vi "计算结果-开启关闭.vi"(5 "油动机试验路径":path=path "D:/研究生/课程/油动机项目/实验文件夹/168-15-6201-004/GV2") -> (0 "计算参数 out":T1, 1 "输入参数":T2, 2 "开启关闭试验":cluster{dbl, dbl, dbl[][]}(graph))   [LabVIEW 2013]
uses:
  <vilib>/Analysis/3filter.llb/Filter Passband Type.ctl
  <vilib>/Utility/config.llb/Read Key (String).vi
  <vilib>/Analysis/3filter.llb/Butterworth Filter (DBL).vi
  <vilib>/Analysis/NI_AALBase.lvlib
  <vilib>/Utility/config.llb/NI_LVConfig.lvlib
panel:
  in  "计算参数 in":T1
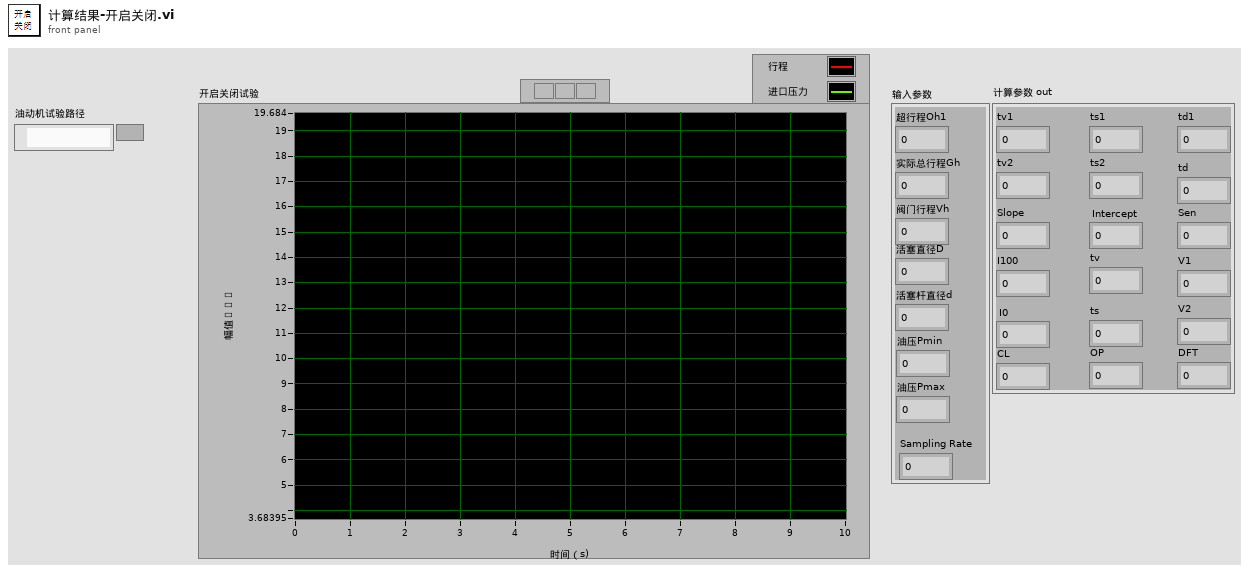
[diagram p1: front panel]
types:
  T1 = cluster{"tv1":dbl, "tv2":dbl, "tv":dbl, "ts1":dbl, "ts2":dbl, "ts":dbl, "td1":dbl, "td":dbl, "Slope":dbl, "Intercept":dbl, "I100":dbl, "I0":dbl, "Sen":dbl, "V1":dbl, "V2":dbl, "CL":dbl, "OP":dbl, "DFT":dbl}
  T2 = cluster{"超行程Oh1":dbl, "实际总行程Gh":dbl, "阀门行程Vh":dbl, "活塞直径D":dbl, "活塞杆直径d":dbl, "油压Pmin":dbl, "油压Pmax":dbl, "Sampling Rate":dbl}
  T3 = typedef "NI_AALBase.lvlib/Filter Passband Type.ctl" = enum32{"Lowpass", "Highpass", "Bandpass", "Bandstop"}
  T4 = typedef "NI_LVConfig.lvlib/Config Data RefNum.ctl" = refnum<k1>
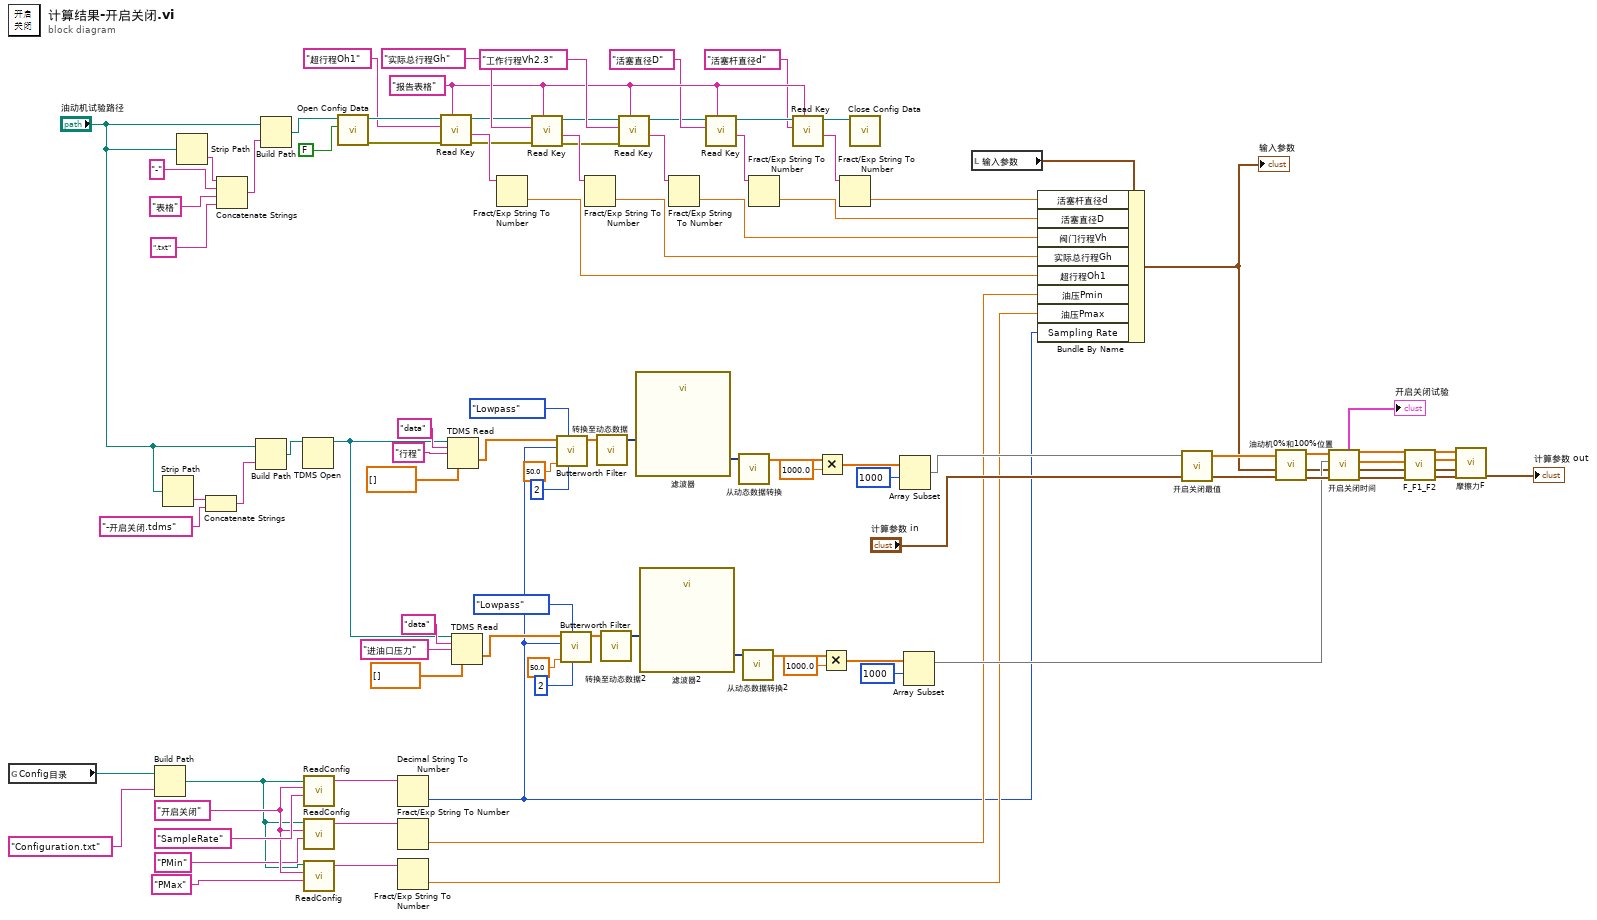
[diagram p0: block diagram]
diagram:
  w17 = "开启关闭" ("Section")
  w54 = "报告表格" ("key")
  n1 = global read "Config目录.vi" "Config目录"() -> (w20:path)
  n2 = Build Path(base path=w20, name or relative path="Configuration.txt") -> (appended path=w14:path)
  n3 = Strip Path(path="油动机试验路径") -> (name=w64:string)  [unwired: 1 out]
  n4 = Strip Path(path="油动机试验路径") -> (name=w61:string)  [unwired: 1 out]
  n5 = Concatenate Strings(w64, "-开启关闭.tdms") -> (w62:string)
  n6 = Concatenate Strings(w61, "-" ("string"), "表格" ("string"), ".txt") -> (w58:string)
  n7 = Build Path(base path="油动机试验路径", name or relative path=w62) -> (appended path=w91:path)
  n8 = Build Path(base path="油动机试验路径", name or relative path=w58) -> (appended path=w57:path)
  n9 = TDMS Open(11:w91) -> (3:w27:refnum<k34>)  [unwired: 6 in, 1 out]
  n10 = call "ReadConfig.vi"("Key"="SampleRate", "Section"=w17, "Path"=w14) -> ("Value"=w23:string)  [unwired: 1 in, 2 out]
  n11 = call "ReadConfig.vi"("Key"="PMin", "Section"=w17, "Path"=w14) -> ("Value"=w19:string)  [unwired: 1 in, 2 out]
  n12 = call "ReadConfig.vi"("Key"="PMax", "Section"=w17, "Path"=w14) -> ("Value"=w18:string)  [unwired: 1 in, 2 out]
  n13 = call <vilib>:"Open Config Data.vi"("create file if necessary (T)"=FALSE, "configuration file path"=w57) -> ("error out"=w90:errorcluster, "refnum"=w89:T4)  [unwired: 7 in, 1 out]
  n14 = Decimal String To Number(string=w23) -> (number=w6:i32)  [unwired: 2 in, 1 out]
  n15 = Fract/Exp String To Number(string=w19) -> (number=w8:dbl)  [unwired: 3 in, 1 out]
  n16 = Fract/Exp String To Number(string=w18) -> (number=w7:dbl)  [unwired: 3 in, 1 out]
  n17 = call-poly <vilib>:"Read Key.vi"("section"=w54, "error in (no error)"=w90, "key"="超行程Oh1", "refnum"=w89) -> ("error out"=w85:errorcluster, "value"=w87:string, "refnum out"=w86:T4)  [unwired: 4 in, 1 out]
  n18 = TDMS Read(0:w27, 5:"data" ("组名称输入"), 7:"行程" ("组名称输入"), 12:dbl[] []) -> (10:w75:dbl[])  [unwired: 4 in, 5 out]
  n19 = TDMS Read(0:w27, 5:"data" ("组名称输入"), 7:"进油口压力" ("组名称输入"), 12:dbl[] []) -> (10:w37:dbl[])  [unwired: 4 in, 5 out]
  n20 = Fract/Exp String To Number(string=w87) -> (number=w46:dbl)  [unwired: 3 in, 1 out]
  n21 = call-poly <vilib>:"Read Key.vi"("section"=w54, "error in (no error)"=w85, "key"="实际总行程Gh", "refnum"=w86) -> ("error out"=w81:errorcluster, "value"=w84:string, "refnum out"=w82:T4)  [unwired: 4 in, 1 out]
  n22 = call-poly <vilib>:"Butterworth Filter.vi"("order"=2, "filter type"=Filter_Passband_Type."Lowpass", "low cutoff freq: fl"=50.0, "sampling freq: fs"=w6, "X"=w75) -> ("Filtered X"=w72:dbl[])  [unwired: 3 in, 1 out]
  n23 = call-poly <vilib>:"Butterworth Filter.vi"("order"=2, "filter type"=Filter_Passband_Type."Lowpass", "low cutoff freq: fl"=50.0, "sampling freq: fs"=w6, "X"=w37) -> ("Filtered X"=w34:dbl[])  [unwired: 3 in, 1 out]
  n24 = Fract/Exp String To Number(string=w84) -> (number=w45:dbl)  [unwired: 3 in, 1 out]
  n25 = call "转换至动态数据"("Array"=w72) -> ("Dynamic Data Type"=w73:dynamicdata)  [unwired: 3 in]
  n26 = call "转换至动态数据2"("Array"=w34) -> ("Dynamic Data Type"=w35:dynamicdata)  [unwired: 3 in]
  n27 = call-poly <vilib>:"Read Key.vi"("section"=w54, "error in (no error)"=w81, "key"="工作行程Vh2.3", "refnum"=w82) -> ("value"=w80:string, "refnum out"=w50:T4)  [unwired: 4 in, 2 out]
  n28 = call "滤波器"("Signal"=w73) -> ("Filtered Signal"=w74:dynamicdata)  [unwired: 9 in, 1 out]
  n29 = call "滤波器2"("Signal"=w35) -> ("Filtered Signal"=w36:dynamicdata)  [unwired: 9 in, 1 out]
  n30 = Fract/Exp String To Number(string=w80) -> (number=w44:dbl)  [unwired: 3 in, 1 out]
  n31 = call-poly <vilib>:"Read Key.vi"("section"=w54, "key"="活塞直径D", "refnum"=w50) -> ("value"=w52:string, "refnum out"=w49:T4)  [unwired: 5 in, 2 out]
  n32 = call "从动态数据转换"("Dynamic Data Type"=w74) -> ("Array"=w78:dbl[])  [unwired: 3 in]
  n33 = call "从动态数据转换2"("Dynamic Data Type"=w36) -> ("Array"=w40:dbl[])  [unwired: 3 in]
  n34 = Fract/Exp String To Number(string=w52) -> (number=w43:dbl)  [unwired: 3 in, 1 out]
  n35 = call-poly <vilib>:"Read Key.vi"("section"=w54, "key"="活塞杆直径d", "refnum"=w49) -> ("value"=w51:string, "refnum out"=w48:T4)  [unwired: 5 in, 2 out]
  n36 = Multiply(x=w78, y=1000.0) -> (x*y=w79:dbl[])
  n37 = Multiply(x=w40, y=1000.0) -> (x*y=w41:dbl[])
  n38 = Fract/Exp String To Number(string=w51) -> (number=w42:dbl)  [unwired: 3 in, 1 out]
  n39 = call <vilib>:"Close Config Data.vi"("refnum"=w48) -> ()  [unwired: 9 in, 2 out]
  n40 = Array Subset(array=w79, index=1000 ("索引")) -> (w96:dbl[])  [unwired: 1 in]
  n41 = Array Subset(array=w41, index=1000 ("索引")) -> (w24:dbl[])  [unwired: 1 in]
  n42 = local read "输入参数"() -> (w92:T2)
  n43 = Bundle By Name(cluster=w92, "活塞杆直径d"=w42, "活塞直径D"=w43, "阀门行程Vh"=w44, "实际总行程Gh"=w45, "超行程Oh1"=w46, "油压Pmin"=w8, "油压Pmax"=w7, "Sampling Rate"=w6) -> (w26:T2)
  "输入参数" <- w26
  n44 = call "开启关闭最值.vi"("计算参数 in"="计算参数 in", "Array in"=w96) -> ("计算参数 out"=w95:T1, "Array out"=w97:dbl[])  [unwired: 2 in]
  n45 = call "油动机0%和100%位置.vi"("计算参数 in"=w95, "输入参数 in"=w26, "Array in"=w97) -> ("计算参数 out"=w98:T1, "输入参数 out"=w5:T2, "Array out"=w11:dbl[])  [unwired: 2 in]
  n46 = call "开启关闭时间.vi"("计算参数 in"=w98, "输入参数 in"=w5, "进口压力信号 in"=w24, "行程 in"=w11) -> ("计算参数 out"=w25:T1, "输入参数 out"=w2:T2, "进口压力信号 out"=w3:dbl[], "行程 out"=w10:dbl[], "Waveform Graph"=→"开启关闭试验":cluster{dbl, dbl, dbl[][]})  [unwired: 1 in]
  n47 = call "F_F1_F2.vi"("计算参数 in"=w25, "输入参数"=w2, "进油口压力数组 in"=w3) -> ("计算参数 out"=w13:T1, "输入参数 out"=w12:T2, "进油口压力数组 out"=w1:dbl[])  [unwired: 4 in]
  n48 = call "摩擦力F.vi"("计算参数 in"=w13, "输入参数"=w12, "进油口压力数组 in"=w1, "行程数组 in"=w10) -> ("计算参数 out"=→"计算参数 out":T1)  [unwired: 5 in, 2 out]
